vi "Config Source.vi"(0 "VISA resource name":refnum<visa-resource-name>, 1 "Autorange (On)":bool=TRUE, 2 "Range (1.000)":dbl=1.0, 3 "Low Range (1.000)":dbl=1.0, 5 "Node In":string, 7 "Channel (Channel A)":T1, 8 "Off Mode (Normal)":u16(ring) items=["Normal", "Zero", "High Z"], 9 "Function (Current)":enum32{"Current", "Voltage"}(ring), 11 "error in":errorcluster, 12 "Level (0.000)":dbl, 13 "Limit (0.1)":dbl=0.1) -> (4 "VISA resource name out":refnum<visa-resource-name>, 6 "Node Out":string, 14 "Command String":string, 15 "error out":errorcluster)   [LabVIEW 2018, in "Keithley 2600 Series.lvlib"]
doc: "This VI will configure a single SMU channel's source.\n\n<b>Note:</b> This VI does not turn the source On/Off. Use Output Enable to turn the source On/Off.\n\n<b>Functions and Attributes Used</b>\nsmuX.source.autorangeY\nsmuX.source.rangeY\nsmuX.source.lowrangeY\nsmuX.source.offmode\nsmuX.source.levelY\nsmuX.source.limitY\nsmuX.source.func"
uses:
  Keithley 2600 Series.lvlib
  Private/GlobalVariables.vi
  Channel.ctl
panel:
  # "(c) 2008 Keithley Instruments, Inc.  ALL RIGHTS RESERVED."
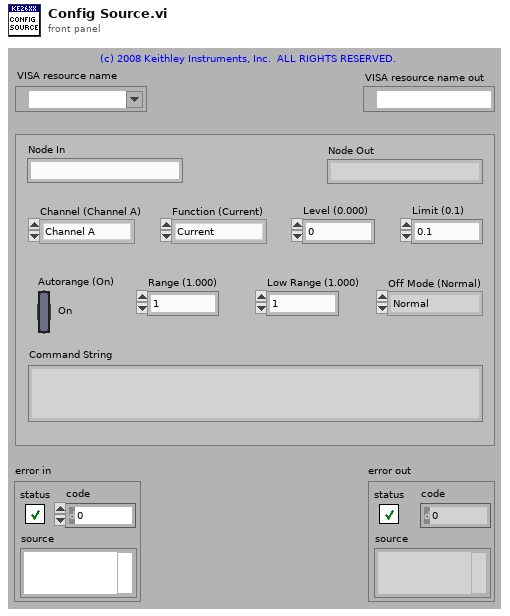
[diagram p1: front panel]
types:
  T1 = typedef "Keithley 2600 Series.lvlib/Channel.ctl" = enum32{"Channel A", "Channel B"}
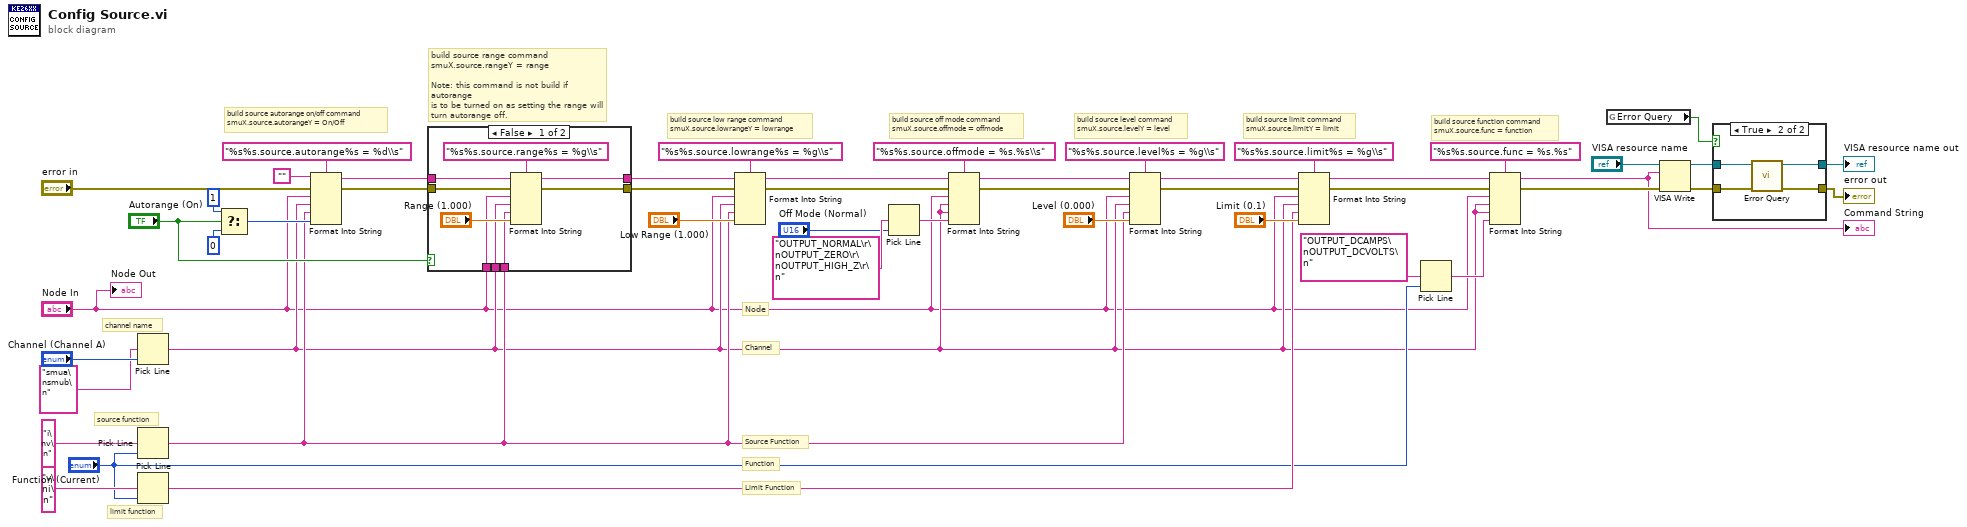
[diagram p0: block diagram]
diagram:
  # "build source function command\nsmuX.source.func = function"
  # "Function"
  # "Limit Function"
  # "Source Function"
  # "Channel"
  # "Node"
  # "build source limit command\nsmuX.source.limitY = limit"
  # "build source level command\nsmuX.source.levelY = level"
  # "build source off mode command\nsmuX.source.offmode = offmode"
  # "build source low range command\nsmuX.source.lowrangeY = lowrange"
  # "build source range command\nsmuX.source.rangeY = range\n\nNote: this command is not build if autorange\nis to be turned on as setting the range will\nturn autorange off."
  # "build source autorange on/off command\nsmuX.source.autorangeY = On/Off"
  # "limit function"
  # "channel name"
  # "source function"
  n1 = Pick Line(multi-line string="smua\nsmub\n", line index="Channel (Channel A)") -> (output string=w6:string)  [unwired: 1 out]
  n2 = Pick Line(multi-line string="i\nv\n", line index="Function (Current)") -> (output string=w11:string)  [unwired: 1 out]
  n3 = Pick Line(multi-line string="v\ni\n", line index="Function (Current)") -> (output string=w26:string)  [unwired: 1 out]
  n4 = Select(t=1, s="Autorange (On)", f=0) -> (s? t:f=w43:i32)
  n5 = Format Into String(format string="%s%s.source.autorange%s = %d\\s", initial string="", error in="error in", "Node In", w6, w11, w43) -> (resulting string=w40:string, error out=w39:errorcluster)
  n6 = case shown="False" "Autorange (On)" {
    tunnel: w40 -> [w56 w60]
    tunnel: w39 -> [w55 w59]
    tunnel: [w54 w59] -> w32
    tunnel: [w53 w60] -> w33
    tunnel: w11 -> [w52 _]
    tunnel: w6 -> [w51 _]
    tunnel: "Node In" -> [w50 _]
    frame False {
      n7 = Format Into String(format string="%s%s.source.range%s = %g\\s", initial string=w56, error in=w55, w50, w51, w52, "Range (1.000)") -> (resulting string=w53:string, error out=w54:errorcluster)
    }
    frame True {
    }
  }
  n8 = Format Into String(format string="%s%s.source.lowrange%s = %g\\s", initial string=w33, error in=w32, "Node In", w6, w11, "Low Range (1.000)") -> (resulting string=w25:string, error out=w22:errorcluster)
  n9 = Pick Line(multi-line string="OUTPUT_NORMAL\r\nOUTPUT_ZERO\r\nOUTPUT_HIGH_Z\r\n" ("options"), line index="Off Mode (Normal)") -> (output string=w31:string)  [unwired: 1 out]
  n10 = Format Into String(format string="%s%s.source.offmode = %s.%s\\s", initial string=w25, error in=w22, "Node In", w6, w6, w31) -> (resulting string=w24:string, error out=w21:errorcluster)
  n11 = Format Into String(format string="%s%s.source.level%s = %g\\s", initial string=w24, error in=w21, "Node In", w6, w11, "Level (0.000)") -> (resulting string=w23:string, error out=w20:errorcluster)
  n12 = Format Into String(format string="%s%s.source.limit%s = %g\\s", initial string=w23, error in=w20, "Node In", w6, w26, "Limit (0.1)") -> (resulting string=w4:string, error out=w3:errorcluster)
  n13 = Pick Line(multi-line string="OUTPUT_DCAMPS\nOUTPUT_DCVOLTS\n", line index="Function (Current)") -> (output string=w7:string)  [unwired: 1 out]
  n14 = Format Into String(format string="%s%s.source.func = %s.%s", initial string=w4, error in=w3, "Node In", w6, w6, w7) -> (resulting string=w1:string, error out=w2:errorcluster)
  "Command String" <- w1
  n15 = global read "GlobalVariables.vi" "Error Query"() -> (w16:bool)
  n16 = VISA Write(VISA resource name="VISA resource name", write buffer=w1, error in (no error)=w2) -> (VISA resource name out=w15:refnum<visa-resource-name>, error out=w14:errorcluster)  [unwired: 1 out]
  n17 = case shown="True" w16 {
    tunnel: w15 -> [w62 w66]
    tunnel: w14 -> [w61 w65]
    tunnel: [w62 w64] -> w13
    tunnel: [w61 w63] -> w12
    frame False {
    }
    frame True {
      n18 = call "Error Query.vi"("error in (no error)"=w65, "VISA resource name"=w66) -> ("error out"=w63:errorcluster, "VISA resource name out"=w64:refnum<visa-resource-name>)  [unwired: 8 out]
    }
  }
  "VISA resource name out" <- w13
  "error out" <- w12
  "Node Out" <- "Node In"
